vi "MARS_IDLE_Cmd.vi"(8 "error in (no error)":errorcluster, 11 "VISA Refnum in":refnum<visa-resource-name>) -> (0 "error out":errorcluster, 3 "VISA Refnum out":refnum<visa-resource-name>)   [LabVIEW 2015]
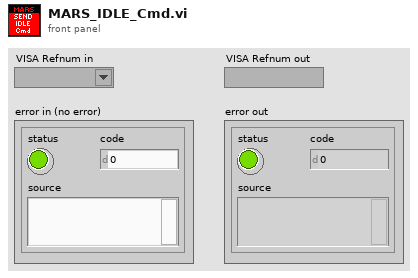
[diagram p1: front panel]
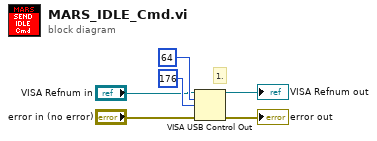
[diagram p0: block diagram]
diagram:
  # "1."
  n1 = VISA USB Control Out(0:"VISA Refnum in", 5:i16 64 ("request type"), 7:i16 176 ("request type"), 11:"error in (no error)") -> (4:→"VISA Refnum out":refnum<visa-resource-name>, 15:→"error out":errorcluster)  [unwired: 3 in]
